vi "Split.vi"(0 "SigMan in":refnum<class "SignalManager.lvclass">, 7 "Name":string, 11 "error in (no error)":errorcluster) -> (4 "SigMan out":refnum<class "SignalManager.lvclass">, 6 "SigMan out 2":refnum<class "SignalManager.lvclass">, 15 "error out":errorcluster)   [LabVIEW 2020, in "SignalManager.lvclass"]
uses:
  SignalManager.lvclass
  SignalManager.lvclass/SignalManager.ctl
  Channel/Channel.lvclass
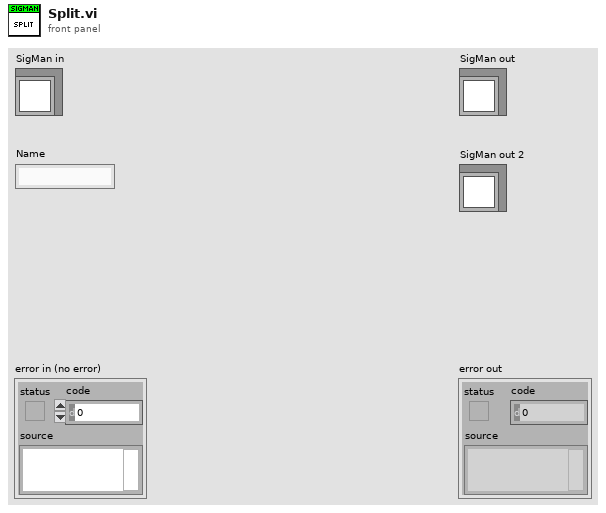
[diagram p1: front panel]
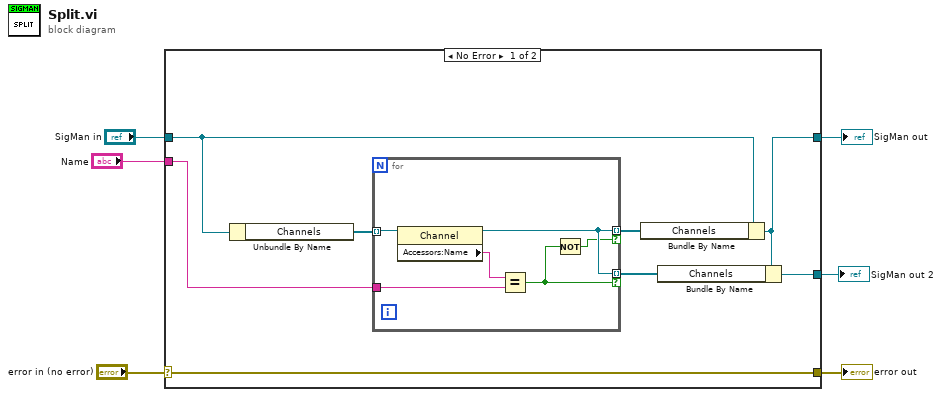
[diagram p0: block diagram]
diagram:
  n1 = case shown="No Error" "error in (no error)" {
    selector: "error in (no error)" -> [w14 w22]
    tunnel: [w14 w22] -> w5
    tunnel: [w9 w21] -> w3
    tunnel: "SigMan in" -> [w11 w21]
    tunnel: "Name" -> [w12 _]
    tunnel: [w7 _] -> w1
    frame No Error {
      n2 = Unbundle By Name(w11) -> ("Channels"=w13:refnum<class "Channel.lvclass">[])
      n3 = for {
        tunnel: w13 -> [w20] mode=indexing
        tunnel: w12 -> [w18]
        tunnel: [w17] -> w10 mode=indexing if=w16
        tunnel: [w17] -> w8 mode=indexing if=w15
        n4 = property class="Channel"(reference=w20) -> (reference out=w17:refnum<class "Channel.lvclass">, "Accessors:Name"=w19:string)  [unwired: 1 in, 1 out]
        n5 = Equal?(x=w19, y=w18) -> (x = y?=w15:bool)
        n6 = Not(x=w15) -> (.not. x?=w16:bool)
      }
      n7 = Bundle By Name(cluster=w11, "Channels"=w10) -> (w9:refnum<class "SignalManager.lvclass">)
      n8 = Bundle By Name(cluster=w9, "Channels"=w8) -> (w7:refnum<class "SignalManager.lvclass">)
    }
    frame Error {
    }
  }
  "error out" <- w5
  "SigMan out" <- w3
  "SigMan out 2" <- w1
